vi "Transmit (I2S).vi"(7 "configuration":T1={"bits per channel"=16, "data set edge"=enum."falling", "invert sync"=FALSE}, 8 "transmit":bool, 9 "input valid":bool, 10 "sample":u32, 11 "clock in":bool) -> (3 "signals out":cluster{"clock":bool, "sync":bool, "sdata":bool}, 4 "ready for input":bool)   [LabVIEW 2013, in "I2S-TDM.lvlib"]
uses:
  I2S-TDM.lvlib
  Controls/i2s transmitter configuration.ctl
  Controls/sync modes.ctl
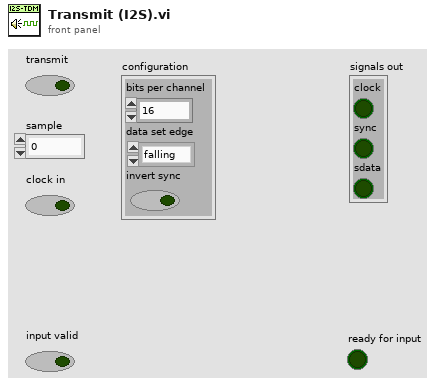
[diagram p1: front panel]
types:
  T1 = typedef "I2S-TDM.lvlib/i2s transmitter configuration.ctl" = cluster{"bits per channel":u8, "data set edge":enum16{"rising", "falling"}, "invert sync":bool}
  T2 = typedef "I2S-TDM.lvlib/sync modes.ctl" = enum16{"Sample Clock", "Pulse"}
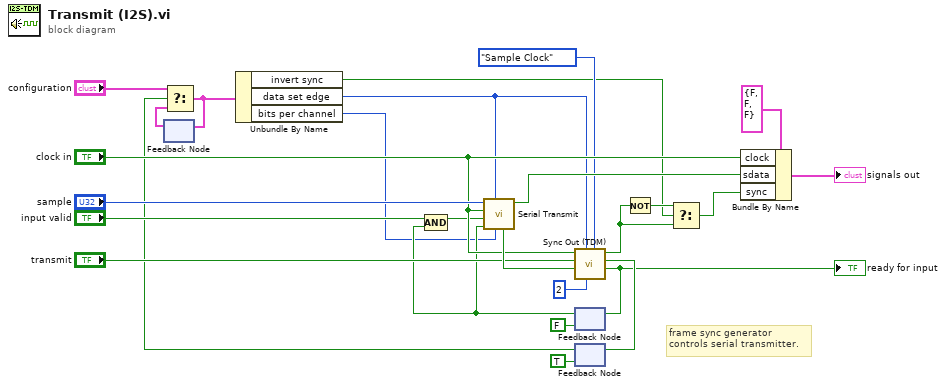
[diagram p0: block diagram]
diagram:
  # "frame sync generator controls serial transmitter."
  n1 = feedback #1() -> (w12:T1)  [unwired: 1 in]
  n2 = feedback #2(FALSE ("ready for input")) -> (w18:bool)
  n3 = Compound Arithmetic op=AND("input valid", w18) -> (w19:bool)
  n4 = feedback #3(TRUE ("ready for input")) -> (w9:bool)
  n5 = Select(t="configuration", s=w9, f=w12) -> (s? t:f=w7:T1)
  n6 = feedback-in #1(w7) -> ()
  n7 = Unbundle By Name(w7) -> ("invert sync"=w2:bool, "data set edge"=w13:enum16{"rising", "falling"}, "bits per channel"=w14:u8)
  n8 = call "Serial Transmit.vi"("transfer length"=w14, "serial clock shift edge (falling)"=w13, "transmit"=w18, "input valid"=w19, "serial clock in"="clock in", "sample"="sample") -> ("data bit out"=w22:bool, "ready for input"=w25:bool)  [unwired: 4 in]
  n9 = call "Sync Out (TDM).vi"("sync mode"=sync_modes."Sample Clock", "channel count (2)"=u8 2, "bit set edge (falling)"=w13, "ready for input?"=w25, "transmit"="transmit", "clock in"="clock in") -> ("ready for input"=w1:bool, "latch config"=w10:bool, "frame sync"=w16:bool)  [unwired: 3 in]
  "ready for input" <- w1
  n10 = feedback-in #2(w1) -> ()
  n11 = feedback-in #3(w10) -> ()
  n12 = Not(x=w16) -> (.not. x?=w17:bool)
  n13 = Select(t=w17, s=w2, f=w16) -> (s? t:f=w15:bool)
  n14 = Bundle By Name(cluster=cluster{"clock":bool, "sync":bool, "sdata":bool} {"clock"=FALSE, "sync"=FALSE, "sdata"=FALSE} ("signals out"), "clock"="clock in", "sdata"=w22, "sync"=w15) -> (→"signals out":cluster{"clock":bool, "sync":bool, "sdata":bool})
